vi "Insert Child.vi"(4 "Position":i32[](array[numeric]), 6 "Tree Item In":T1, 8 "error in (no error)":errorcluster, 9 "Data In":refnum<class "Tree Data.lvclass">, 10 "Tree In":refnum<class "Tree.lvclass">, 11 "Composite Tree Data in":refnum<class "Composite Tree Data.lvclass">) -> (0 "error out":errorcluster, 2 "Tree Out":refnum<class "Tree.lvclass">, 3 "Composite Tree Data out":refnum<class "Composite Tree Data.lvclass">)   [LabVIEW 2024, in "Composite Tree Data.lvclass"]
uses:
  Composite Tree Data.lvclass
  Tree Data/Tree Data.lvclass
  Tree/Tree.lvclass
  Tree/Type Def/Tree Item.ctl
  Tree Data/Tree Data.lvclass/Tree Data.ctl
  Tree/Tree.lvclass/Tree.ctl
  Composite Tree Data.lvclass/Composite Tree Data.ctl
  Tree/Public Data/Read Root Tag.vi
  Tree Data/Protected Data/Read Tag.vi
  Polymorphic VIs/Tree Converter/Tag To BFS Index.vi
  Polymorphic VIs/Tree Converter/BFS Index To Tag.vi
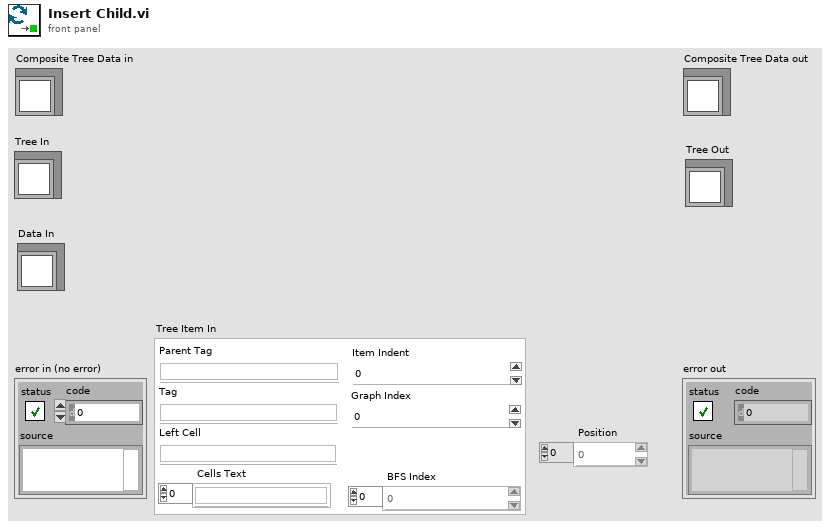
[diagram p1: front panel]
types:
  T1 = typedef "Tree Item.ctl" = cluster{"Parent Tag":string, "Tag":string, "Left Cell":string, "Cells Text":string[], "BFS Index":i32[], "Graph Index":i32, "Item Indent":i32}
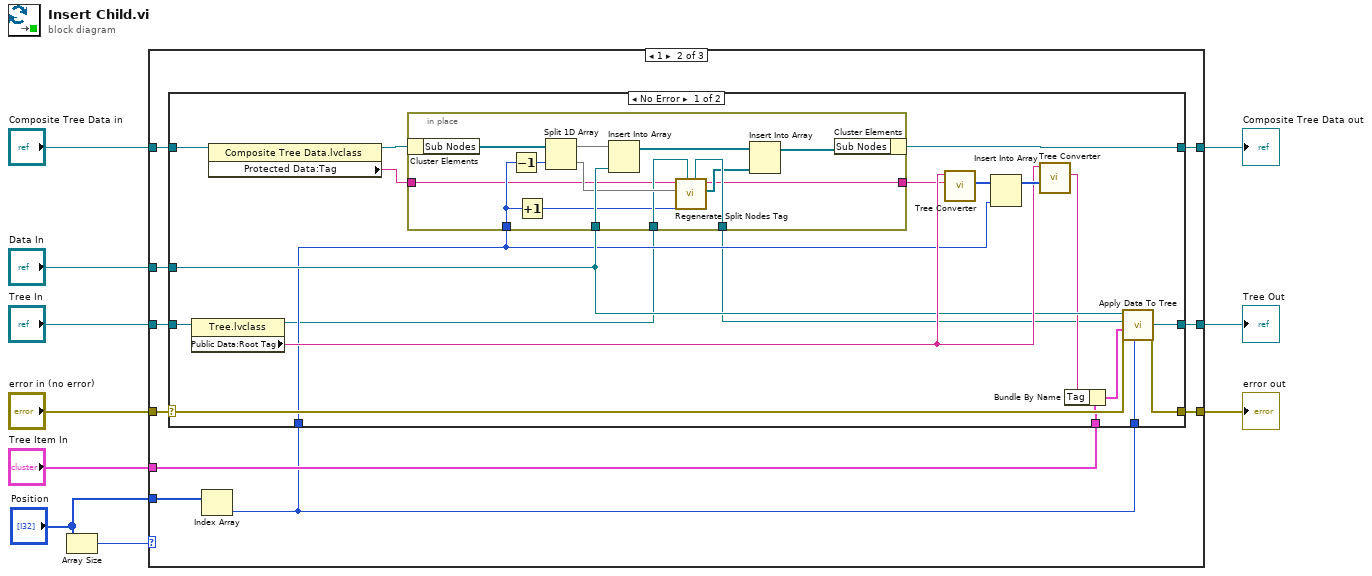
[diagram p0: block diagram]
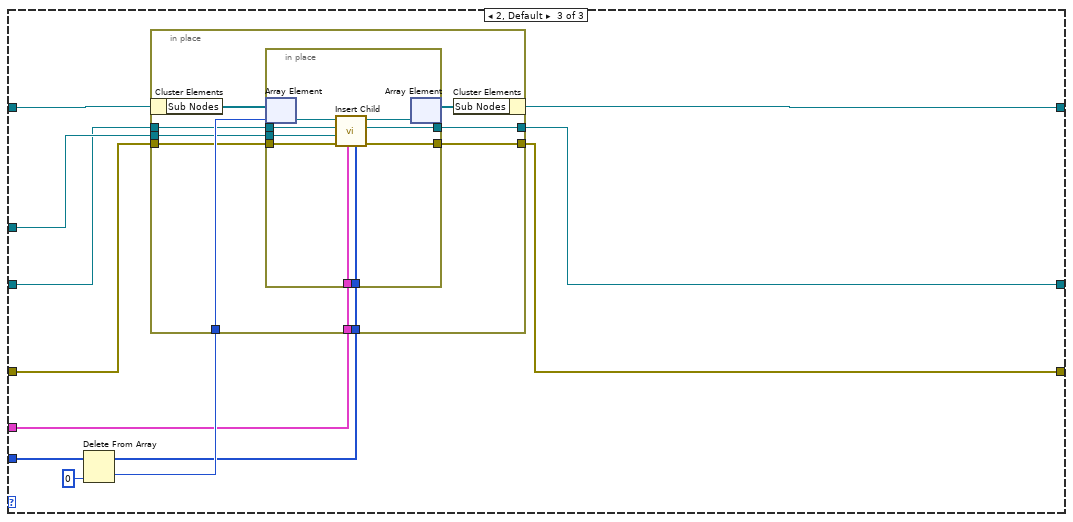
[diagram p4: hidden frame]
diagram:
  n1 = Array Size(array="Position") -> (size(s)=w2:i32)
  n2 = case shown="1" w2 {
    tunnel: "error in (no error)" -> [w11 w23 w65]
    tunnel: [w11 w22 w61] -> w9
    tunnel: "Composite Tree Data in" -> [w13 w21 w69]
    tunnel: [w13 w20 w68] -> w7
    tunnel: "Data In" -> [_ w19 w67]
    tunnel: [w12 w18 w62] -> w5
    tunnel: "Tree In" -> [w12 w17 w66]
    tunnel: "Tree Item In" -> [_ w16 w64]
    tunnel: "Position" -> [_ w15 w63]
    frame 0 {
    }
    frame 1 {
      n3 = Index Array(array=w15) -> (element=w14:i32)  [unwired: 1 in]
      n4 = case shown="No Error" w23 {
        selector: w23 -> [w38 w60]
        tunnel: [w36 w60] -> w22
        tunnel: [w28 w59] -> w20
        tunnel: w21 -> [w27 w59]
        tunnel: w19 -> [w37 _]
        tunnel: [w39 w58] -> w18
        tunnel: w17 -> [w43 w58]
        tunnel: w16 -> [w35 _]
        tunnel: w14 -> [w32 _]
        tunnel: w14 -> [w31 _]
        frame No Error {
          n5 = property class="Tree.lvclass"(reference=w43) -> (reference out=w30:refnum<class "Tree.lvclass">, "Public Data:Root Tag"=w40:string)  [unwired: 1 in, 1 out]
          n6 = property class="Composite Tree Data.lvclass"(reference=w27) -> (reference out=w26:refnum<class "Composite Tree Data.lvclass">, "Protected Data:Tag"=w25:string)  [unwired: 1 in, 1 out]
          n7 = in-place {
            in-place-border: w37 -> [w55]
            in-place-border: w32 -> [w47]
            in-place-border: w30 -> [w52]
            in-place-border: [w51] -> w29
            in-place-border: w25 -> [w45]
            in-place-border: [w44] -> w24
            n8 = in-place-cluster #1(w26) -> ("Sub Nodes"=w57:refnum<class "Tree Data.lvclass">[])
            n9 = Decrement(x=w47) -> (x-1=w54:i32)
            n10 = Increment(x=w47) -> (x+1=w46:i32)
            n11 = Split 1D Array(array=w57, index=w54) -> (first subarray=w56:refnum<class "Tree Data.lvclass">[], second subarray=w53:refnum<class "Tree Data.lvclass">[])
            n12 = Insert Into Array(array=w56, new element=w55) -> (w50:refnum<class "Tree Data.lvclass">[])  [unwired: 1 in]
            n13 = call "Regenerate Split Nodes Tag.vi"("Tree In"=w52, "Start Index"=w46, "Split Node In"=w53, "Parent Tag In"=w45) -> ("Split Node Out"=w48:refnum<class "Tree Data.lvclass">[], "Parent Tag Out"=w44:string, "Tree Out"=w51:refnum<class "Tree.lvclass">)  [unwired: 5 in]
            n14 = Insert Into Array(array=w50, new element=w48) -> (w49:refnum<class "Tree Data.lvclass">[])  [unwired: 1 in]
            n15 = in-place-cluster #1("Sub Nodes"=w49) -> (w28:refnum<class "Composite Tree Data.lvclass">)
          }
          n16 = call-poly "Tree Converter.vi"("Tag In"=w24, "Root Tag"=w40) -> ("BFS Index Out"=w42:i32[])  [unwired: 9 in]
          n17 = Insert Into Array(array=w42, new element=w32) -> (w41:i32[])  [unwired: 1 in]
          n18 = call-poly "Tree Converter.vi"("BFS Index In"=w41, "Root Tag In"=w40) -> ("Tag Out"=w34:string)  [unwired: 9 in]
          n19 = Bundle By Name(cluster=w35, "Tag"=w34) -> (w33:T1)
          n20 = call-dynamic "Apply Data To Tree.vi"("Child Position"=w31, "error in (no error)"=w38, "Tree Item In"=w33, "Tree In"=w29, "Tree Data in"=w37) -> ("error out"=w36:errorcluster, "Tree Out"=w39:refnum<class "Tree.lvclass">)  [unwired: 4 in, 1 out]
        }
        frame Error {
        }
      }
    }
    frame 2, Default {
      n21 = Delete From Array(array=w63, index=0) -> (deleted portion=w71:i32, array with subset deleted=w70:i32[])  [unwired: 1 in]
      n22 = in-place {
        in-place-border: w71 -> [w81]
        in-place-border: w66 -> [w79]
        in-place-border: w65 -> [w78]
        in-place-border: w67 -> [w77]
        in-place-border: w64 -> [w76]
        in-place-border: w70 -> [w75]
        in-place-border: [w74] -> w62
        in-place-border: [w73] -> w61
        n23 = in-place-cluster #2(w69) -> ("Sub Nodes"=w82:refnum<class "Tree Data.lvclass">[])
        n24 = in-place {
          in-place-border: w79 -> [w89]
          in-place-border: w78 -> [w87]
          in-place-border: w77 -> [w88]
          in-place-border: w76 -> [w86]
          in-place-border: w75 -> [w85]
          in-place-border: [w84] -> w74
          in-place-border: [w83] -> w73
          n25 = in-place-array #3(w82, w81) -> (w91:refnum<class "Tree Data.lvclass">)
          n26 = call-dynamic "Insert Child.vi"("Position"=w85, "Tree Item In"=w86, "error in (no error)"=w87, "Data In"=w88, "Tree In"=w89, "Tree Data in"=w91) -> ("error out"=w83:errorcluster, "Tree Out"=w84:refnum<class "Tree.lvclass">, "Tree Data out"=w90:refnum<class "Tree Data.lvclass">)  [unwired: 3 in]
          n27 = in-place-array #3(w90) -> (w80:refnum<class "Tree Data.lvclass">[])  [unwired: 1 out]
        }
        n28 = in-place-cluster #2("Sub Nodes"=w80) -> (w68:refnum<class "Composite Tree Data.lvclass">)
      }
    }
  }
  "error out" <- w9
  "Composite Tree Data out" <- w7
  "Tree Out" <- w5
